vi "Init WebView2 Core.vi"(8 "error in (no error)":errorcluster, 11 "WebView2":refnum<class "WebView2 Control.lvclass">) -> (0 "error out":errorcluster, 3 "WebView2.lvlib:WebView2 Control.lvclass":refnum<class "WebView2 Control.lvclass">)   [LabVIEW 2020, in "WebView2.lvlib" / "WebView2 Control.lvclass"]
uses:
  WebView2 Control.lvclass
  WebView2 Control.lvclass/WebView2 Control.ctl
  C:/Users/Simon/Documents/GitHub/LV-WebView2/Source/Libs/Microsoft.Web.WebView2.WinForms.dll
  Libs/Microsoft.Web.WebView2.WinForms.dll
  C:/Users/Simon/Documents/GitHub/LV-WebView2/Source/Libs/Microsoft.Web.WebView2.Core.dll
  Libs/Microsoft.Web.WebView2.Core.dll
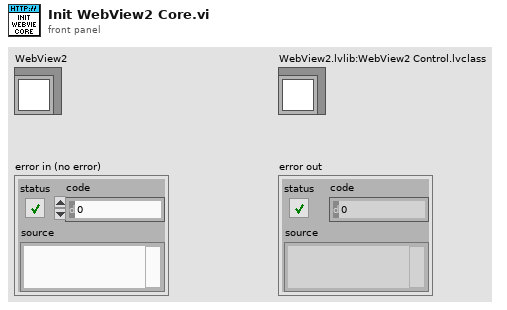
[diagram p1: front panel]
types:
  T1 = typedef "WebView2.lvlib/WebView2 Control.lvclass/Res.ctl" = cluster{"WebView2":refnum<k24>, "Webview2 Core":refnum<k24>, "event callback":refnum<k27>, "Environment":refnum<k24>}
  T2 = typedef "WebView2.lvlib/WebView2 Control.lvclass/Paths.ctl" = cluster{"Webview2 Native":path, "Edge Application":path, "User Data":path}
  T3 = typedef "WebView2.lvlib/WebView2 Control.lvclass/Core Env Options.ctl" = cluster{"additionalBrowserArguments":string, "language":string, "targetCompatibleBrowserVersion":string, "allowSingleSignOnUsingOSPrimaryAccount":bool}
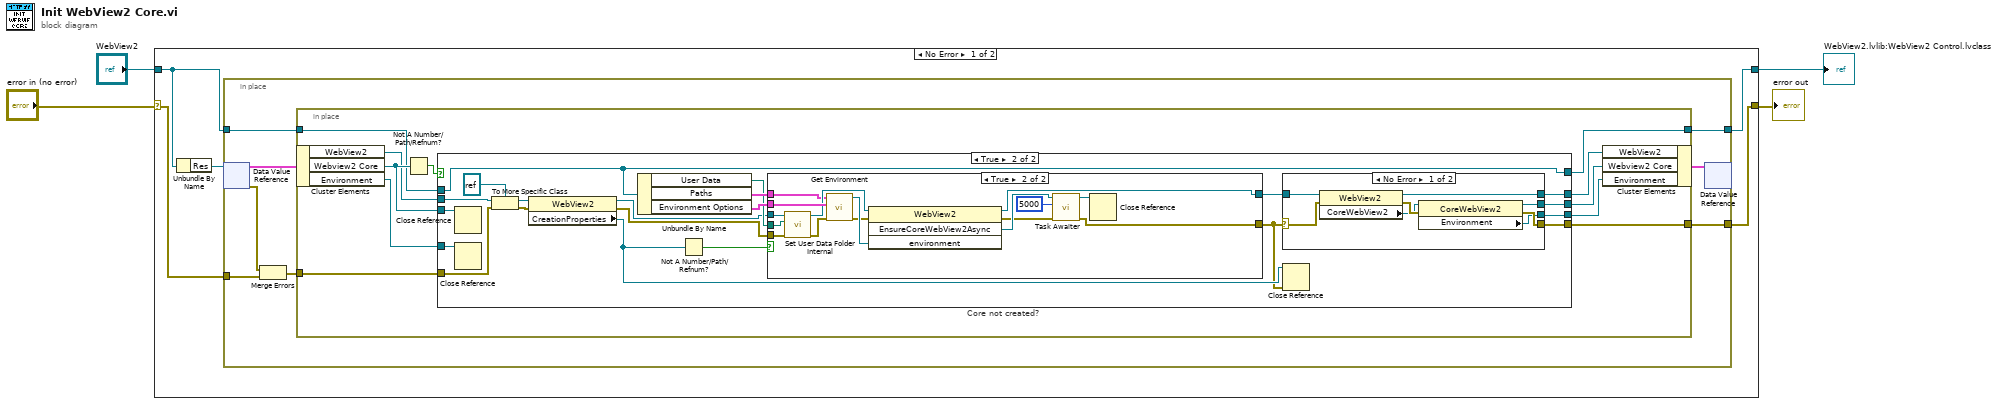
[diagram p0: block diagram]
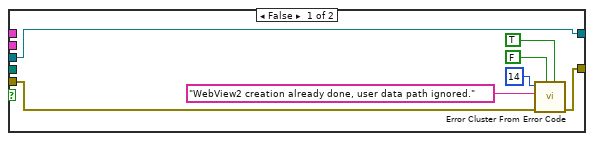
[diagram p3: hidden frame]
diagram:
  n1 = case shown="No Error" "error in (no error)" {
    selector: "error in (no error)" -> [w8 w88]
    tunnel: [w9 w88] -> w4
    tunnel: [w5 w87] -> w2
    tunnel: "WebView2" -> [w6 w87]
    frame No Error {
      n2 = Unbundle By Name(w6) -> ("Res"=w7:refnum<data-value>)
      n3 = in-place {
        in-place-border: [w17] -> w9
        in-place-border: w6 -> [w16]
        in-place-border: w8 -> [w15]
        in-place-border: [w10] -> w5
        n4 = in-place-dvr #1(w7) -> (w14:T1, w11:errorcluster)
        n5 = Merge Errors(w11, w15) -> (w12:errorcluster)
        n6 = in-place {
          in-place-border: [w27] -> w17
          in-place-border: w12 -> [w24]
          in-place-border: w16 -> [w21]
          in-place-border: [w18] -> w10
          n7 = in-place-cluster #2(w14) -> ("WebView2"=w25:refnum<k24>, "Webview2 Core"=w26:refnum<k24>, "Environment"=w19:refnum<k24>)
          n8 = Not A Number/Path/Refnum?(number/path/refnum=w26) -> (NaN/Path/Refnum?=w28:bool)
          n9 = case "Core not created?" shown="True" w28 {
            tunnel: [w33 w50] -> w22
            tunnel: w26 -> [w33 w49]
            tunnel: w25 -> [w31 w47]
            tunnel: w24 -> [w32 w41]
            tunnel: [w32 w51] -> w27
            tunnel: [w31 w53] -> w23
            tunnel: w21 -> [w29 w44]
            tunnel: [w30 w48] -> w20
            tunnel: w19 -> [w30 w45]
            tunnel: [w29 w44] -> w18
            frame False {
            }
            frame True {
              n10 = Close Reference(reference=w49) -> ()  [unwired: 1 in, 1 out]
              n11 = Close Reference(reference=w45) -> ()  [unwired: 1 in, 1 out]
              n12 = To More Specific Class(target class=refnum<k24> refnum ("Webview2"), reference=w47, error in=w41) -> (specific class reference=w39:refnum<k24>, error out=w40:errorcluster)
              n13 = property class="WebView2"(reference=w39, error in=w40) -> (reference out=w38:refnum<k24>, error out=w36:errorcluster, "CreationProperties"=w35:refnum<k24>)
              n14 = Unbundle By Name(w44) -> ("User Data"=w43:path, "Paths"=w46:T2, "Environment Options"=w52:T3)
              n15 = Not A Number/Path/Refnum?(number/path/refnum=w35) -> (NaN/Path/Refnum?=w37:bool)
              n16 = case shown="True" w37 {
                tunnel: [w55 w76] -> w54
                tunnel: w52 -> [_ w75]
                tunnel: [w56 w74] -> w34
                tunnel: w46 -> [_ w72]
                tunnel: w43 -> [_ w71]
                tunnel: w36 -> [w57 w69]
                tunnel: w38 -> [w55 w68]
                frame False {
                  n17 = call <vilib>:"Error Cluster From Error Code.vi"("is warning? (False)"=TRUE, "show call chain? (False)"=FALSE, "error in (no error)"=w57, "error message (\"\")"="WebView2 creation already done, user data path ignored." ("error message (\"\")"), "error code (0)"=14) -> ("error out"=w56:errorcluster)  [unwired: 4 in]
                }
                frame True {
                  n18 = call "Set User Data Folder Internal.vi"("error in (no error)"=w69, "User Data"=w71, "Webview2"=w68) -> ("error out"=w70:errorcluster, "Webview2"=w73:refnum<k24>)  [unwired: 7 in]
                  n19 = call "Get Environment.vi"("error in"=w70, 10:w75, "Paths"=w72) -> ("error out"=w62:errorcluster, "Environment out"=w64:refnum<k24>)  [unwired: 7 in]
                  n20 = invoke class="WebView2" method="EnsureCoreWebView2Async"(reference=w73, error in=w62, "environment"=w64) -> (reference out=w76:refnum<k24>, error out=w63:errorcluster, "EnsureCoreWebView2Async"=w67:refnum<k24>)  [unwired: 1 in, 1 out]
                  n21 = call "Task Awaiter.vi"("error in (no error)"=w63, "Timeout"=5000, "Task"=w67) -> ("error out"=w74:errorcluster, "Task"=w65:refnum<k24>)  [unwired: 6 in, 1 out]
                  n22 = Close Reference(reference=w65) -> ()  [unwired: 1 in, 1 out]
                }
              }
              n23 = case shown="No Error" w34 {
                selector: w34 -> [w82 w85]
                tunnel: w54 -> [w84 w86]
                tunnel: [w78 _] -> w50
                tunnel: [w83 w86] -> w53
                tunnel: [w80 w85] -> w51
                tunnel: [w77 _] -> w48
                frame No Error {
                  n24 = property class="WebView2"(reference=w84, error in=w82) -> (reference out=w83:refnum<k24>, error out=w81:errorcluster, "CoreWebView2"=w79:refnum<k24>)
                  n25 = property class="CoreWebView2"(reference=w79, error in=w81) -> (reference out=w78:refnum<k24>, error out=w80:errorcluster, "Environment"=w77:refnum<k24>)
                }
                frame Error {
                }
              }
              n26 = Close Reference(reference=w35, error in (no error)=w34) -> ()  [unwired: 1 out]
            }
          }
          n27 = in-place-cluster #2("WebView2"=w23, "Webview2 Core"=w22, "Environment"=w20) -> (w13:T1)
        }
        n28 = in-place-dvr #1(w13) -> ()  [unwired: 2 out]
      }
    }
    frame Error {
    }
  }
  "error out" <- w4
  "WebView2.lvlib:WebView2 Control.lvclass" <- w2
